vi "GV Nframes.vi"() -> ()   [LabVIEW 2017]
panel:
  out "Nframes":i16
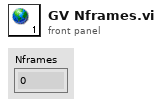
[diagram p1: front panel]
diagram:
